vi "Check Unit of Work.vi"(8 "error in (no error)":errorcluster, 11 "Entity Manager in":refnum<class "Entity Manager.lvclass">) -> (0 "error out":errorcluster, 3 "Entity Manager out":refnum<class "Entity Manager.lvclass">, 5 "Unit Of Work":refnum<class "Unit Of Work Session.lvclass">)   [LabVIEW 2020, in "Conditu2.lvlib" / "Entity Manager.lvclass"]
uses:
  Entity Manager.lvclass
  Unit Of Work Session/Unit Of Work Session.lvclass
  Entity Manager.lvclass/Entity Manager.ctl
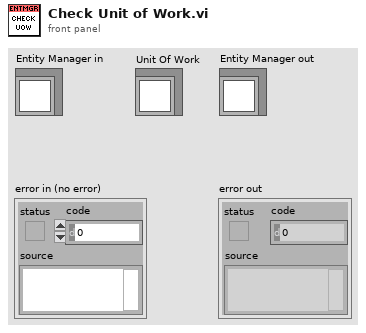
[diagram p1: front panel]
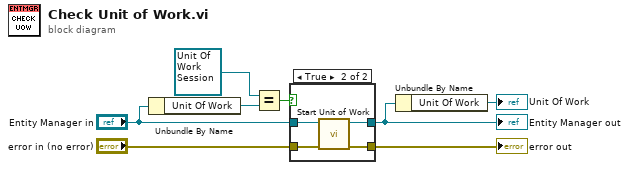
[diagram p0: block diagram]
diagram:
  n1 = Unbundle By Name("Entity Manager in") -> ("Unit Of Work"=w3:refnum<class "Unit Of Work Session.lvclass">)
  n2 = Equal?(x=refnum<class "Unit Of Work Session.lvclass"> refnum ("y"), y=w3) -> (x = y?=w7:bool)
  n3 = case shown="True" w7 {
    tunnel: "Entity Manager in" -> [w9 w14]
    tunnel: [w9 w13] -> w2
    tunnel: "error in (no error)" -> [w10 w12]
    tunnel: [w10 w11] -> w5
    frame False {
    }
    frame True {
      n4 = call "Start Unit of Work.vi"("error in (no error)"=w12, "Entity Manager in"=w14) -> ("error out"=w11:errorcluster, "Entity Manager out"=w13:refnum<class "Entity Manager.lvclass">)  [unwired: 8 in]
    }
  }
  "error out" <- w5
  "Entity Manager out" <- w2
  n5 = Unbundle By Name(w2) -> ("Unit Of Work"=→"Unit Of Work":refnum<class "Unit Of Work Session.lvclass">)
